vi "H2O und CO2 umrechnen.vi"(11 "Aktuelle Messwerte":sgl[](array[numeric])) -> (3 "Aktuelle Messwerte":sgl[](array[numeric]))   [LabVIEW 2020, in "AK-Schnittstelle.lvlib"]
uses:
  AK-Schnittstelle.lvlib
  Seiten/FT-IR/FGV FT-IR Gasliste Aktionen.ctl
  Allgemein/allgemeine Sub-VIs.lvlib
  Seiten/FT-IR/FT-IR.lvlib
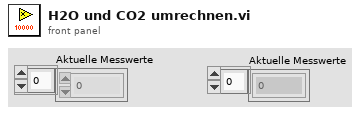
[diagram p1: front panel]
types:
  T1 = typedef "FT-IR.lvlib/FGV FT-IR Gasliste Aktionen.ctl" = enum16{"lesen", "Gasliste FT-IR", "Gasliste ausgelesen", "laden", "speichern", "löschen"}
  T2 = typedef "String - Ausgabefeld.ctl" = string
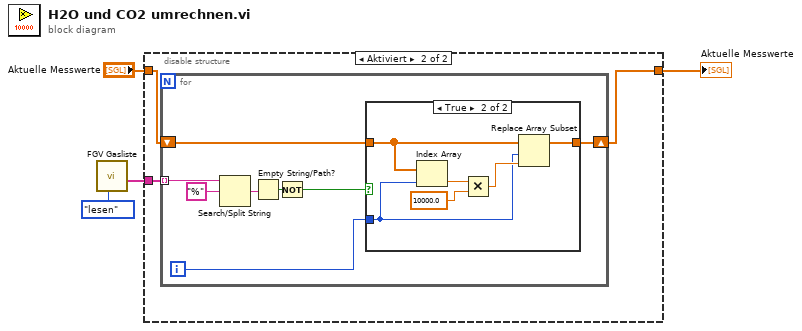
[diagram p0: block diagram]
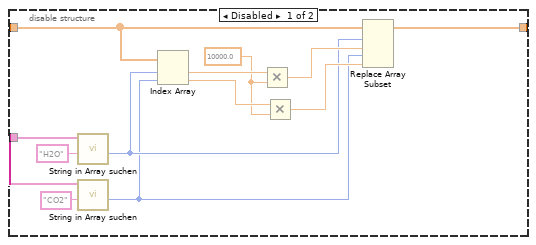
[diagram p2: hidden frame]
diagram:
  n1 = call "FGV Gasliste.vi"("Aktionen"=FGV_FT-IR_Gasliste_Aktionen."lesen") -> ("Aktuelle Gasliste gesamt"=w3:T2[])  [unwired: 8 in, 2 out]
  n2 = disable-structure shown="Aktiviert" {
    disable-tunnel: w3 -> [w16 w19]
    disable-tunnel: "Aktuelle Messwerte" -> [w13 w18]
    disable-tunnel: [w5 w17] -> w1
    frame Disabled {
      w10 = sgl 10000.0 ("y")
      n3 = call "String in Array suchen.vi"("Nach String/Zeichen suchen (-)"="H2O", "String-Array"=w16) -> ("Index"=w7:i32)  [unwired: 8 in, 1 out]
      n4 = call "String in Array suchen.vi"("Nach String/Zeichen suchen (-)"="CO2", "String-Array"=w16) -> ("Index"=w6:i32)  [unwired: 8 in, 1 out]
      n5 = Index Array(array=w13, index #1=w7, index #2=w6) -> (element #1=w12:sgl, element #2=w11:sgl)
      n6 = Multiply(x=w12, y=w10) -> (x*y=w9:sgl)
      n7 = Multiply(x=w11, y=w10) -> (x*y=w8:sgl)
      n8 = Replace Array Subset(array=w13, new element #1=w9, index #1=w7, new element #2=w8, index #2=w6) -> (w5:sgl[])
    }
    frame Enabled {
      n9 = for {
        tunnel: w19 -> [w20] mode=indexing
        shift-right: [w27] -> w17
        shift-left: w18 -> [w26]
        i -> [w22]
        n10 = Search/Split String(string=w20, search string/char (-)="%" ("Nach String/Zeichen suchen (-)")) -> (match + rest of string=w23:T2)  [unwired: 1 in, 2 out]
        n11 = Empty String/Path?(string/path=w23) -> (empty?=w24:bool)
        n12 = Not(x=w24) -> (.not. x?=w21:bool)
        n13 = case shown="True" w21 {
          tunnel: w22 -> [_ w32]
          tunnel: [w28 w31] -> w27
          tunnel: w26 -> [w28 w30]
          frame False {
          }
          frame True {
            n14 = Index Array(array=w30, index=w32) -> (element=w29:sgl)
            n15 = Multiply(x=w29, y=sgl 10000.0) -> (x*y=w33:sgl)
            n16 = Replace Array Subset(array=w30, new element=w33, index=w32) -> (w31:sgl[])
          }
        }
      }
    }
  }
  "Aktuelle Messwerte" <- w1
